vi "Simulated Serial Instrument.vi"() -> ()   [LabVIEW 2020, in "VISA Measurement.lvlib"]
uses:
  VISA Measurement.lvlib
  <vilib>/Instr/_visa.llb/VISA Configure Serial Port (Instr).vi
panel:
  in  "stop":bool
  in  "VISA resource name":refnum<visa-resource-name>
  out "error out":errorcluster
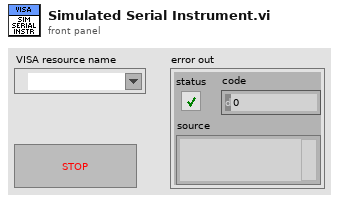
[diagram p1: front panel]
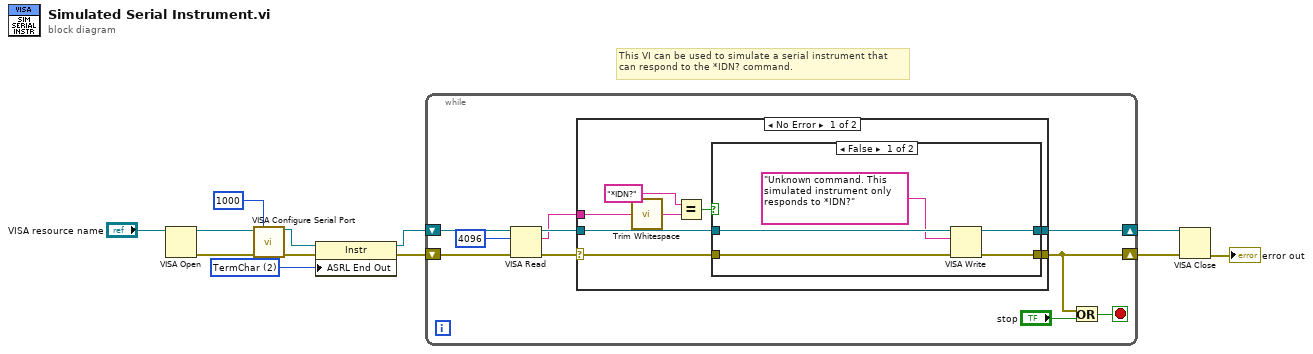
[diagram p0: block diagram]
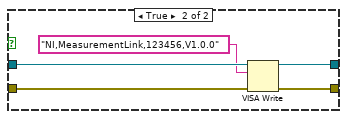
[diagram p2: hidden frame]
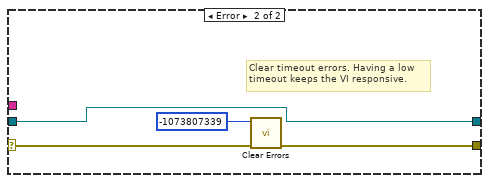
[diagram p3: hidden frame]
diagram:
  w1 = u16 2 items=["None", "Last Bit", "TermChar", "Break"] ("Serial Settings:End Mode for Writes")
  # "This VI can be used to simulate a serial instrument that \ncan respond to the *IDN? command."
  n1 = VISA Open(VISA resource name="VISA resource name") -> (VISA resource name=w7:refnum<visa-resource-name>, error out=w8:errorcluster)  [unwired: 4 in]
  n2 = call-poly "VISA Configure Serial Port"("VISA resource name"=w7, "timeout (10sec)"=u32 1000, "error in (no error)"=w8) -> ("VISA resource name out"=w3:refnum<visa-resource-name>, "error out"=w5:errorcluster)  [unwired: 11 in]
  n3 = property class="Instr"(reference=w3, error in=w5, "ASRL End Out"=w1) -> (reference out=w2:refnum<visa-resource-name>, error out=w4:errorcluster)
  n4 = while {
    shift-right: [w15] -> w10
    shift-left: w2 -> [w21]
    shift-right: [w14] -> w11
    shift-left: w4 -> [w20]
    stop <- w19 stop-if-true
    n5 = VISA Read(VISA resource name=w21, byte count=u32 4096, error in (no error)=w20) -> (VISA resource name out=w16:refnum<visa-resource-name>, read buffer=w13:string, error out=w17:errorcluster)  [unwired: 1 out]
    n6 = case shown="No Error" w17 {
      selector: w17 -> [w30 w44]
      tunnel: w16 -> [w29 w41]
      tunnel: [w28 w41] -> w15
      tunnel: [w27 w42] -> w14
      tunnel: w13 -> [w25 _]
      frame No Error {
        n7 = call <vilib>:"Trim Whitespace.vi"("string"=w25) -> ("trimmed string"=w26:string)  [unwired: 1 in]
        n8 = Equal?(x="*IDN?", y=w26) -> (x = y?=w23:bool)
        n9 = case shown="False" w23 {
          tunnel: w30 -> [w35 w40]
          tunnel: w29 -> [w34 w39]
          tunnel: [w33 w38] -> w28
          tunnel: [w32 w37] -> w27
          frame False {
            n10 = VISA Write(VISA resource name=w34, write buffer="Unknown command. This simulated instrument only responds to *IDN?", error in (no error)=w35) -> (VISA resource name out=w33:refnum<visa-resource-name>, error out=w32:errorcluster)  [unwired: 1 out]
          }
          frame True {
            n11 = VISA Write(VISA resource name=w39, write buffer="NI,MeasurementLink,123456,V1.0.0", error in (no error)=w40) -> (VISA resource name out=w38:refnum<visa-resource-name>, error out=w37:errorcluster)  [unwired: 1 out]
          }
        }
      }
      frame Error {
        # "Clear timeout errors. Having a low\ntimeout keeps the VI responsive."
        n12 = call <vilib>:"Clear Errors.vi"("error in (no error)"=w44, "specific error code to clear (0: all)"=-1073807339) -> ("error out"=w42:errorcluster)  [unwired: 4 in, 1 out]
      }
    }
    n13 = Or(x=w14, y="stop") -> (x .or. y?=w19:bool)
  }
  n14 = VISA Close(VISA resource name=w10, error in (no error)=w11) -> (error out=→"error out":errorcluster)
